vi "Read mods.vi"(8 "error in":errorcluster, 11 "modification container in":refnum<class "modification container.lvclass">) -> (0 "error out":errorcluster, 2 "mods":refnum<class "VI modification.lvclass">[](array[class]), 3 "modification container out":refnum<class "modification container.lvclass">)   [LabVIEW 2013, in "modification container.lvclass"]
uses:
  modification container.lvclass
  VI modification.lvclass
  modification container.lvclass/modification container.ctl
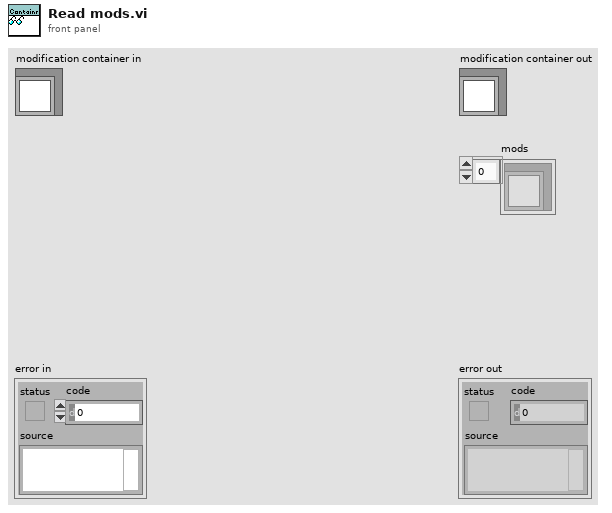
[diagram p1: front panel]
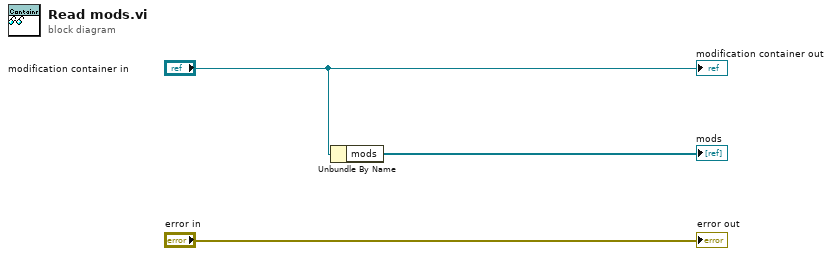
[diagram p0: block diagram]
diagram:
  n1 = Unbundle By Name("modification container in") -> ("mods"=→"mods":refnum<class "VI modification.lvclass">[])
  "error out" <- "error in"
  "modification container out" <- "modification container in"
